vi "G#Object_Clear.vi"(5 "error in (no error)":errorcluster) -> (19 "error out":errorcluster)   [LabVIEW 2020, in "G#Object.lvclass"]
doc: "Clears all remaining queues and events used by the G# object lists. It also kills all class attributes queues and data value references as well as the external create process (if running)."
uses:
  G#Object.lvclass
  utils/G#Object_State.ctl
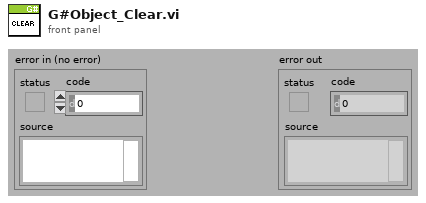
[diagram p1: front panel]
types:
  T1 = cluster{"queue name":string, "reference":refnum<class "G#Object.lvclass">}
  T2 = cluster{"queue name":string, "reference":refnum<class "G#Object.lvclass">}[]
  T3 = cluster{cluster{"queue name":string, "reference":refnum<class "G#Object.lvclass">}[]}[]
  T4 = cluster{string, "reference":refnum<class "G#Object.lvclass">}
  T5 = cluster{string, "reference":refnum<class "G#Object.lvclass">}[]
  T6 = cluster{cluster{string, "reference":refnum<class "G#Object.lvclass">}[]}[]
  T7 = typedef "G#Object.lvclass/G#Object_State.ctl" = enum16{"Clear", "Create", "Delete", "Get class attributes", "Class hierarchy", "Get attribute value", "Set attribute value"}
  T8 = cluster{cluster{"queue name":string, "reference":refnum<class "G#Object.lvclass">}[]}
  T9 = cluster{cluster{string, "reference":refnum<class "G#Object.lvclass">}[]}
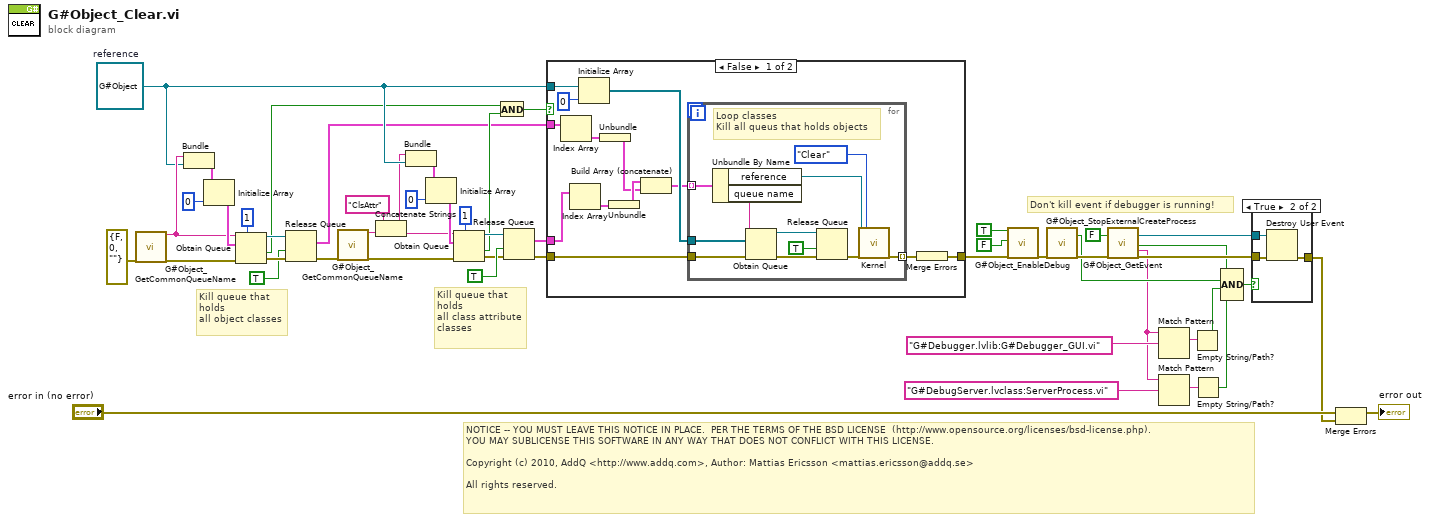
[diagram p0: block diagram]
diagram:
  w9 = refnum<class "G#Object.lvclass"> refnum  # reference
  # "Kill queue that\nholds\nall class attribute\nclasses"
  # "NOTICE -- YOU MUST LEAVE THIS NOTICE IN PLACE.  PER THE TERMS OF THE BSD LICENSE  (http://www.opensource.org/licenses/bsd-license.php).\nYOU MAY SUBLICENSE THIS SOFTWARE IN ANY WAY THAT DOES NOT CONFLICT WITH THIS LICENSE.\n\nCopyright (c) 2010, AddQ <http://www.addq.com>, Author: Mattias Ericsson <mattias.ericsson@addq.se>\n\nAll rights reserved."
  # "Don't kill event if debugger is running!"
  # "Kill queue that\nholds\nall object classes"
  n1 = call "G#Object_GetCommonQueueName.vi"("error in (no error)"=errorcluster {"status"=FALSE, "code"=0, "source"=""}) -> ("queue name"=w27:string, "error out"=w28:errorcluster)  [unwired: 17 in]
  n2 = Bundle("queue name"=w27, "reference"=w9) -> (w44:T1)  [unwired: 1 in]
  n3 = Initialize Array(w44, 0 ("dimension size")) -> (w43:T2)
  n4 = Obtain Queue(max queue size (-1, unlimited)=1, name (unnamed)=w27, element data type=w43, error in (no error)=w28) -> (queue out=w49:refnum<queue>, created new?=w8:bool, error out=w50:errorcluster)  [unwired: 1 in]
  n5 = Release Queue(queue=w49, force destroy? (F)=TRUE, error in (no error)=w50) -> (remaining elements=w4:T3, error out=w5:errorcluster)  [unwired: 1 out]
  n6 = call "G#Object_GetCommonQueueName.vi"("error in (no error)"=w5) -> ("queue name"=w19:string, "error out"=w2:errorcluster)  [unwired: 17 in]
  n7 = Concatenate Strings("ClsAttr" ("string"), w19) -> (w3:string)
  n8 = Bundle(w3, "reference"=w9) -> (w15:T4)  [unwired: 1 in]
  n9 = Initialize Array(w15, 0 ("dimension size")) -> (w16:T5)
  n10 = Obtain Queue(max queue size (-1, unlimited)=1, name (unnamed)=w3, element data type=w16, error in (no error)=w2) -> (queue out=w12:refnum<queue>, created new?=w7:bool, error out=w11:errorcluster)  [unwired: 1 in]
  n11 = And(x=w8, y=w7) -> (x .and. y?=w6:bool)
  n12 = Release Queue(queue=w12, force destroy? (F)=TRUE, error in (no error)=w11) -> (remaining elements=w1:T6, error out=w10:errorcluster)  [unwired: 1 out]
  n13 = case shown="False" w6 {
    tunnel: w10 -> [w62 w75]
    tunnel: [w59 w75] -> w31
    tunnel: w9 -> [w58 _]
    tunnel: w4 -> [w61 _]
    tunnel: w1 -> [w55 _]
    frame False {
      n14 = Index Array(array=w61) -> (element=w60:T8)  [unwired: 1 in]
      n15 = Index Array(array=w55) -> (element=w54:T9)  [unwired: 1 in]
      n16 = Initialize Array(w58, 0 ("dimension size")) -> (w57:refnum<class "G#Object.lvclass">[])
      n17 = Unbundle(w60) -> (w51:T2)
      n18 = Unbundle(w54) -> (w52:T5)
      n19 = Build Array (concatenate)(w52, w51) -> (w53:T2)
      n20 = for {
        tunnel: [w66] -> w63 mode=indexing
        tunnel: w62 -> [w71]
        tunnel: w57 -> [w70]
        tunnel: w53 -> [w69] mode=indexing
        # "Loop classes\nKill all queus that holds objects"
        n21 = Unbundle By Name(w69) -> ("reference"=w65:refnum<class "G#Object.lvclass">, "queue name"=w68:string)
        n22 = Obtain Queue(name (unnamed)=w68, element data type=w70, error in (no error)=w71) -> (queue out=w74:refnum<queue>, error out=w73:errorcluster)  [unwired: 2 in, 1 out]
        n23 = Release Queue(queue=w74, force destroy? (F)=TRUE, error in (no error)=w73) -> (error out=w67:errorcluster)  [unwired: 2 out]
        n24 = call-dynamic "Kernel.vi"("reference in"=w65, "error in (no error)"=w67, "state"=G#Object_State."Clear" ("State")) -> ("error out"=w66:errorcluster)  [unwired: 8 in, 8 out]
      }
      n25 = Merge Errors(w63) -> (w59:errorcluster)
    }
    frame True {
    }
  }
  n26 = call "G#Object_EnableDebug.vi"("set (F)"=TRUE, "debug enable (F)"=FALSE, "error in (no error)"=w31) -> ("error out"=w32:errorcluster)  [unwired: 14 in, 2 out]
  n27 = call "G#Object_StopExternalCreateProcess.vi"("error in (no error)"=w32) -> ("stopped?"=w30:bool, "error out"=w35:errorcluster)  [unwired: 17 in]
  n28 = call "G#Object_GetEvent.vi"("create if needed (T)"=FALSE ("CreateIfNeeded"), "error in (no error)"=w35) -> ("G# event"=w41:refnum<user-event>, "valid"=w38:bool, "event owner"=w25:string, "error out"=w40:errorcluster)  [unwired: 13 in, 1 out]
  n29 = Match Pattern(string=w25, regular expression="G#Debugger.lvlib:G#Debugger_GUI.vi") -> (match substring=w23:string)  [unwired: 1 in, 3 out]
  n30 = Match Pattern(string=w25, regular expression="G#DebugServer.lvclass:ServerProcess.vi") -> (match substring=w21:string)  [unwired: 1 in, 3 out]
  n31 = Empty String/Path?(string/path=w23) -> (empty?=w22:bool)
  n32 = Empty String/Path?(string/path=w21) -> (empty?=w20:bool)
  n33 = Compound Arithmetic op=AND(w38, w30, w22, w20) -> (w37:bool)
  n34 = case shown="True" w37 {
    tunnel: w40 -> [w76 w79]
    tunnel: [w76 w77] -> w36
    tunnel: w41 -> [_ w78]
    frame False {
    }
    frame True {
      n35 = Destroy User Event(user event=w78, error in=w79) -> (error out=w77:errorcluster)
    }
  }
  n36 = Merge Errors("error in (no error)", w36) -> (→"error out":errorcluster)
